vi "IHL_Wait for Start Pos Helper.vi"(8 "error in (no error)":errorcluster, 10 "Inspect Helper Loop Data":T1={"IHL State"=enum."Init", "Timeout"=0, "Loop Count"=0, "Start Sample No."=0, "Collecting Data"=FALSE, "No. Samples"=0, "Success Flag"=FALSE, "Inspect Status "={"Ready"=FALSE, "Inspecting"=FALSE, "Cancel"=FALSE}, "Status"=0, "Encoder Count"=0, "PosToStartScan"=50800, "ScanLength"=50800, "MaxSamples"=50800, "PosToEndScan"=0, "Host SampleData"=refnum, "data value reference"=refnum, "Block Cnt notifier out"=refnum, "EventLog"=refnum}, 11 "Message Queue in":refnum<class "Delacor_lib_QMH_Message Queue.lvclass">) -> (0 "error out":errorcluster, 2 "Inspect Helper Loop Data out":T1={"IHL State"=enum."Init", "Timeout"=0, "Loop Count"=0, "Start Sample No."=0, "Collecting Data"=FALSE, "No. Samples"=0, "Success Flag"=FALSE, "Inspect Status "={"Ready"=FALSE, "Inspecting"=FALSE, "Cancel"=FALSE}, "Status"=0, "Encoder Count"=0, "PosToStartScan"=50800, "ScanLength"=50800, "MaxSamples"=50800, "PosToEndScan"=0, "Host SampleData"=refnum, "data value reference"=refnum, "Block Cnt notifier out"=refnum, "EventLog"=refnum})   [LabVIEW 2015, in "Tool Module.lvlib"]
uses:
  Tool Module.lvlib
  _IHL Data Cluster--typedef.ctl
  Event Logger Library/Event Log/EventLog.lvclass
  _IHL SM Enum--typedef.ctl
  _IHL Status Update Cluster--typedef.ctl
  _Sample Data Rtn Cluster--typedef.ctl
  <vilib>/Delacor/Delacor QMH/Libraries/Message Queue_class/Delacor_lib_QMH_Message Queue.lvclass
  <vilib>/Delacor/Delacor QMH/Libraries/Message Queue_class/Delacor_lib_QMH_Message Queue.lvclass/Delacor_lib_QMH_Message Queue.ctl
  <vilib>/Delacor/Delacor QMH/Libraries/Message Queue_class/Delacor_lib_QMH_Enqueue Message (Single).vi
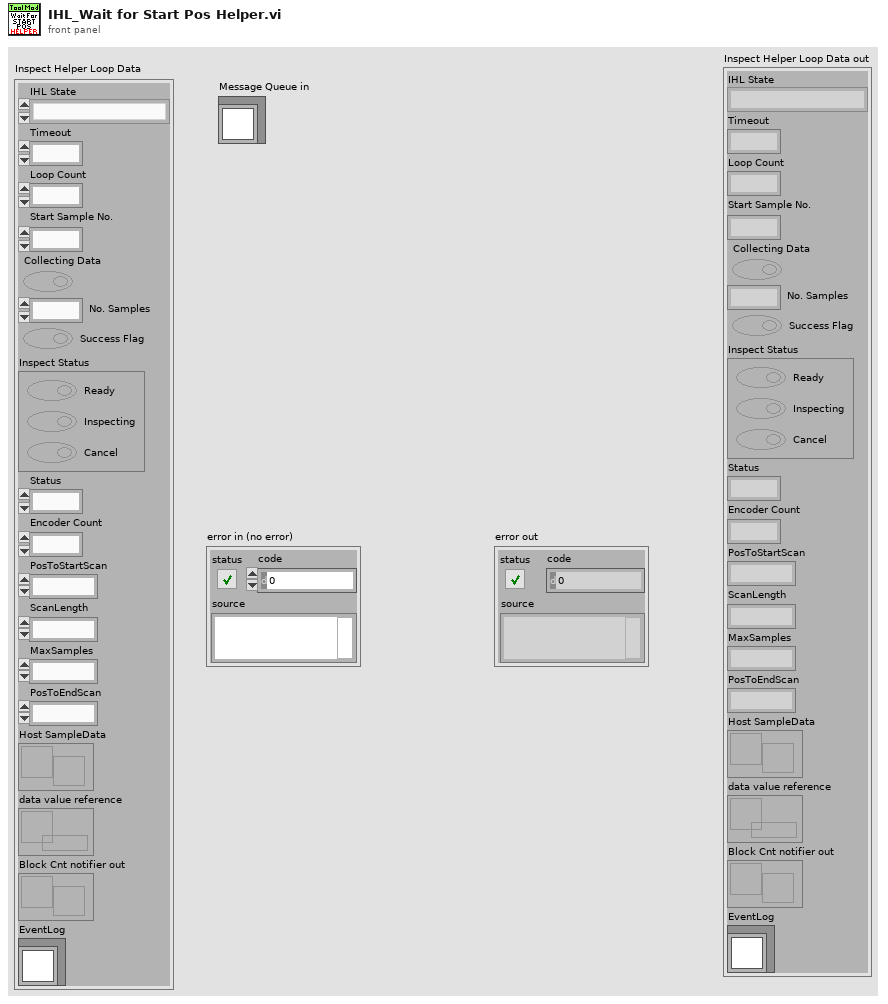
[diagram p1: front panel]
types:
  T1 = typedef "Tool Module.lvlib/_IHL Data Cluster--typedef.ctl" = cluster{"IHL State":T2, "Timeout":i32, "Loop Count":i32, "Start Sample No.":u32, "Collecting Data":bool, "No. Samples":i32, "Success Flag":bool, "Inspect Status ":T3, "Status":u16, "Encoder Count":i32, "PosToStartScan":i32, "ScanLength":i32, "MaxSamples":i32, "PosToEndScan":i32, "Host SampleData":refnum<notifier>, "data value reference":refnum<data-value>, "Block Cnt notifier out":refnum<notifier>, "EventLog":refnum<class "EventLog.lvclass">}
  T2 = typedef "Tool Module.lvlib/_IHL SM Enum--typedef.ctl" = enum16{"Init", "Set Motion Speed", "Move To Scan Start", "Wait for Motion Out", "Wait for Start Pos", "Inspect: START", "Wait for Motion IN", "Wait for Inspect Range", "Inspecting", "Inspect: STOP"}
  T3 = typedef "Tool Module.lvlib/_IHL Status Update Cluster--typedef.ctl" = cluster{"Ready":bool, "Inspecting":bool, "Cancel":bool}
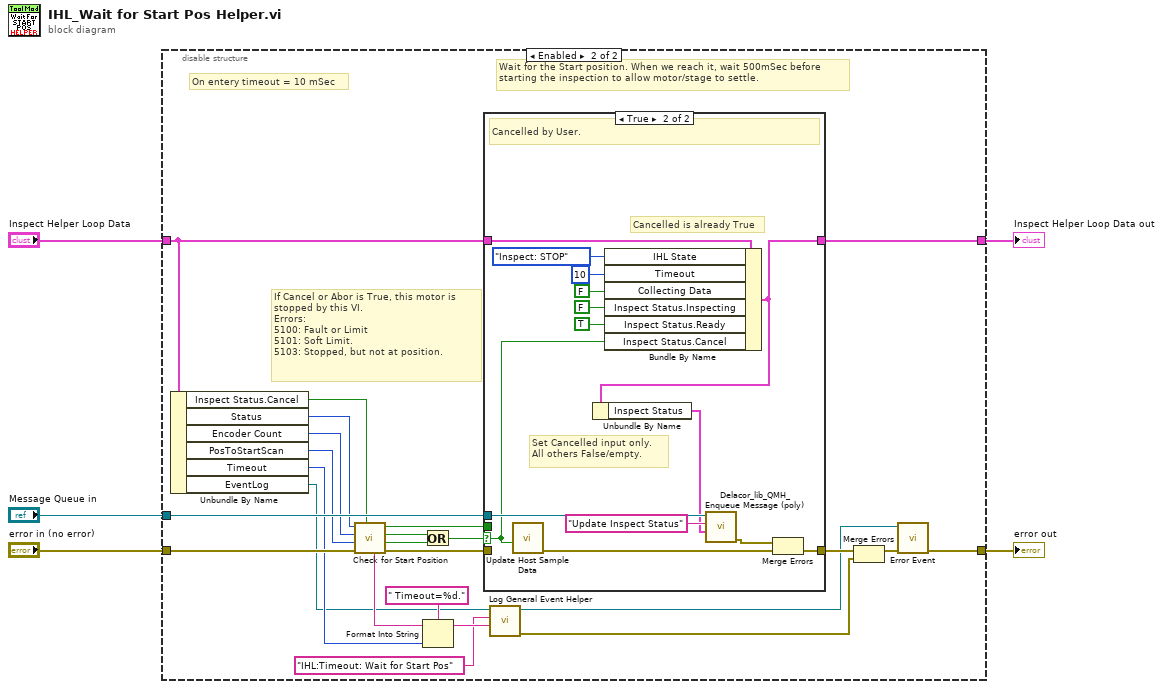
[diagram p0: block diagram]
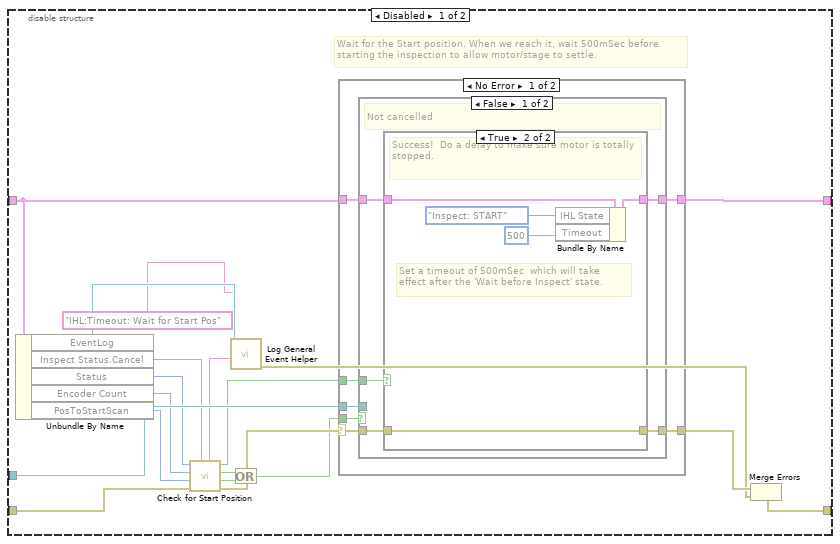
[diagram p2: hidden frame]
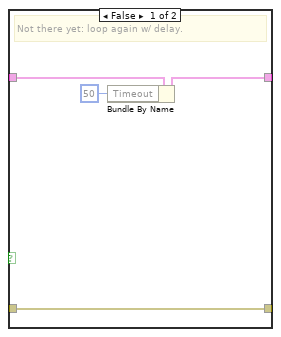
[diagram p3: hidden frame]
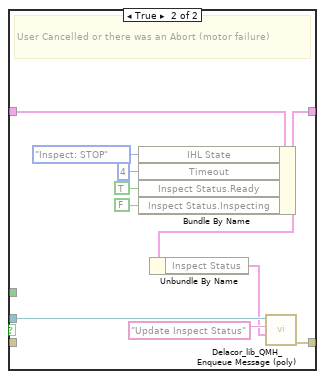
[diagram p4: hidden frame]
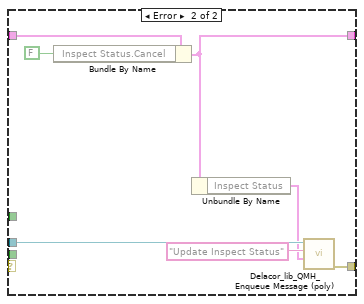
[diagram p5: hidden frame]
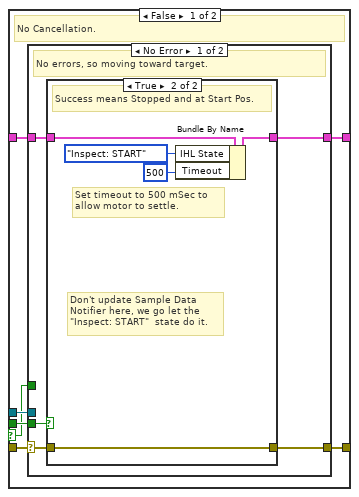
[diagram p6: hidden frame]
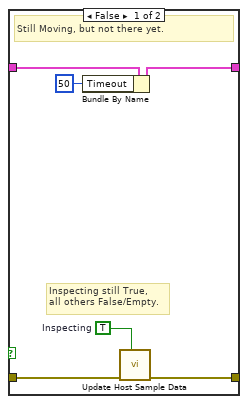
[diagram p7: hidden frame]
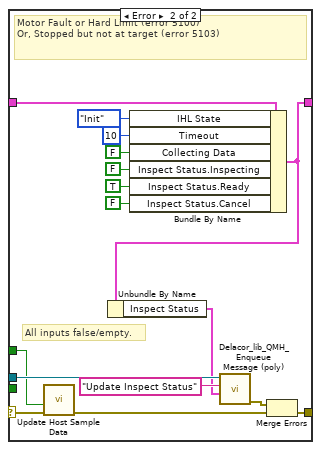
[diagram p8: hidden frame]
diagram:
  n1 = disable-structure shown="Enabled" {
    disable-tunnel: "Message Queue in" -> [w23 w80]
    disable-tunnel: "error in (no error)" -> [w18 w78]
    disable-tunnel: "Inspect Helper Loop Data" -> [w17 w81]
    disable-tunnel: [w11 w82] -> w2
    disable-tunnel: [w7 w72] -> w1
    frame Disabled {
      # "Wait for the Start position. When we reach it, wait 500mSec before starting the inspection to allow motor/stage to settle."
      n2 = Unbundle By Name(w17) -> ("EventLog"=w10:refnum<class "EventLog.lvclass">, "Inspect Status.Cancel"=w22:bool, "Status"=w21:u16, "Encoder Count"=w20:i32, "PosToStartScan"=w19:i32)
      n3 = call "Check for Start Position.vi"("Cancel Inspect"=w22, "error in (no error)"=w18, "Target Encdr Pos."=w19, "Cur Encoder Value"=w20, "Status Byte"=w21) -> ("error out"=w24:errorcluster, "Aborted"=w16:bool, "Cancelled"=w15:bool, "Success"=w13:bool, "Log String out"=w9:string)  [unwired: 2 in]
      n4 = call "Log General Event Helper.vi"("Payload"=w9, "State Info"="IHL:Timeout: Wait for Start Pos", "EventLog in"=w10) -> ("error out"=w6:errorcluster)  [unwired: 7 in, 1 out]
      n5 = Or(x=w15, y=w16) -> (x .or. y?=w14:bool)
      n6 = case shown="No Error" w24 {
        selector: w24 -> [w25 _]
        tunnel: [w31 w60] -> w12
        tunnel: w23 -> [w30 w59]
        tunnel: w17 -> [w29 w62]
        tunnel: [w28 w57] -> w11
        tunnel: w14 -> [w27 _]
        tunnel: w13 -> [w26 _]
        frame No Error {
          n7 = case shown="False" w27 {
            tunnel: [w32 w55] -> w31
            tunnel: w30 -> [_ w54]
            tunnel: w29 -> [w34 w52]
            tunnel: [w33 w51] -> w28
            tunnel: w26 -> [w36 _]
            tunnel: w25 -> [w35 _]
            frame False {
              # "Not cancelled"
              n8 = case shown="True" w36 {
                tunnel: w35 -> [w37 w41]
                tunnel: w34 -> [w40 w45]
                tunnel: [w39 w44] -> w33
                tunnel: [w37 w41] -> w32
                frame False {
                  # "Not there yet: loop again w/ delay."
                  n9 = Bundle By Name(cluster=w40, "Timeout"=50) -> (w39:T1)
                }
                frame True {
                  # "Set a timeout of 500mSec  which will take effect after the 'Wait before Inspect' state."
                  # "Success!  Do a delay to make sure motor is totally stopped."
                  n10 = Bundle By Name(cluster=w45, "IHL State"=_IHL_SM_Enum--typedef."Inspect: START" ("Inspect State"), "Timeout"=500) -> (w44:T1)
                }
              }
            }
            frame True {
              # "User Cancelled or there was an Abort (motor failure)"
              n11 = Bundle By Name(cluster=w52, "IHL State"=_IHL_SM_Enum--typedef."Inspect: STOP" ("Inspect State"), "Timeout"=4, "Inspect Status.Ready"=TRUE ("Inspect Status .Ready"), "Inspect Status.Inspecting"=FALSE ("Inspect Status .Inspecting")) -> (w51:T1)
              n12 = Unbundle By Name(w51) -> ("Inspect Status"=w48:T3)
              n13 = call-poly <vilib>:"Delacor_lib_QMH_Enqueue Message (poly).vi"("Message Data"=w48, "Message"="Update Inspect Status", "Message Queue in"=w54) -> ("error out"=w55:errorcluster)  [unwired: 7 in, 1 out]
            }
          }
        }
        frame Error {
          n14 = Bundle By Name(cluster=w62, "Inspect Status.Cancel"=FALSE ("Inspect Status .Cancel")) -> (w57:T1)
          n15 = Unbundle By Name(w57) -> ("Inspect Status"=w56:T3)
          n16 = call-poly <vilib>:"Delacor_lib_QMH_Enqueue Message (poly).vi"("Message Data"=w56, "Message"="Update Inspect Status", "Message Queue in"=w59) -> ("error out"=w60:errorcluster)  [unwired: 7 in, 1 out]
        }
      }
      n17 = Merge Errors(w12, w6) -> (w7:errorcluster)
    }
    frame Enabled {
      # "If Cancel or Abor is True, this motor is stopped by this VI.\nErrors: \n5100: Fault or Limit\n5101: Soft Limit. \n5103: Stopped, but not at position."
      # "On entery timeout = 10 mSec"
      # "Wait for the Start position. When we reach it, wait 500mSec before starting the inspection to allow motor/stage to settle."
      n18 = Unbundle By Name(w81) -> ("Inspect Status.Cancel"=w66:bool, "Status"=w67:u16, "Encoder Count"=w77:i32, "PosToStartScan"=w76:i32, "Timeout"=w69:i32, "EventLog"=w68:refnum<class "EventLog.lvclass">)
      n19 = call "Check for Start Position.vi"("Cancel Inspect"=w66, "error in (no error)"=w78, "Target Encdr Pos."=w76, "Cur Encoder Value"=w77, "Status Byte"=w67) -> ("error out"=w75:errorcluster, "Aborted"=w65:bool, "Cancelled"=w64:bool, "Success"=w74:bool, "Log String out"=w70:string)  [unwired: 2 in]
      n20 = Or(x=w64, y=w65) -> (x .or. y?=w63:bool)
      n21 = Format Into String(format string=" Timeout=%d.", initial string=w70, w69) -> (resulting string=w85:string)  [unwired: 1 in, 1 out]
      n22 = case shown="True" w63 {
        selector: w63 -> [w87 w126]
        tunnel: [w92 w131] -> w82
        tunnel: w81 -> [w93 w139]
        tunnel: w80 -> [w89 w133]
        tunnel: [w90 w128] -> w79
        tunnel: w75 -> [w91 _]
        tunnel: w74 -> [w88 _]
        frame False {
          # "No Cancellation."
          n23 = case shown="No Error" w91 {
            selector: w91 -> [w95 w114]
            tunnel: w93 -> [w97 w125]
            tunnel: [w96 w118] -> w92
            tunnel: [w94 w111] -> w90
            tunnel: w89 -> [_ w120]
            tunnel: w88 -> [w98 _]
            tunnel: w87 -> [_ w113]
            frame No Error {
              # "No errors, so moving toward target."
              n24 = case shown="True" w98 {
                tunnel: [w103 w108] -> w96
                tunnel: w97 -> [w104 w109]
                tunnel: w95 -> [w100 w105]
                tunnel: [w99 w105] -> w94
                frame False {
                  w101 = TRUE  # Inspecting
                  # "Inspecting still True,\nall others False/Empty."
                  # "Still Moving, but not there yet."
                  n25 = Bundle By Name(cluster=w104, "Timeout"=50) -> (w103:T1)
                  n26 = call "Update Host Sample Data.vi"("Inspecting"=w101, "error in (no error)"=w100) -> ("error out"=w99:errorcluster)  [unwired: 9 in]
                }
                frame True {
                  # "Don't update Sample Data Notifier here, we go let the  \"Inspect: START\"  state do it."
                  # "Set timeout to 500 mSec to allow motor to settle."
                  # "Success means Stopped and at Start Pos."
                  n27 = Bundle By Name(cluster=w109, "IHL State"=_IHL_SM_Enum--typedef."Inspect: START" ("Inspect State"), "Timeout"=500) -> (w108:T1)
                }
              }
            }
            frame Error {
              # "All inputs false/empty."
              # "Motor Fault or Hard Limit (error 5100)\nOr, Stopped but not at target (error 5103)"
              n28 = call "Update Host Sample Data.vi"("error in (no error)"=w114, "Cancelled"=w113) -> ("error out"=w110:errorcluster)  [unwired: 9 in]
              n29 = Bundle By Name(cluster=w125, "IHL State"=_IHL_SM_Enum--typedef."Init" ("Inspect State"), "Timeout"=10, "Collecting Data"=FALSE, "Inspect Status.Inspecting"=FALSE ("Inspect Status .Inspecting"), "Inspect Status.Ready"=TRUE ("Inspect Status .Ready"), "Inspect Status.Cancel"=FALSE ("Inspect Status .Cancel")) -> (w118:T1)
              n30 = Unbundle By Name(w118) -> ("Inspect Status"=w117:T3)
              n31 = call-poly <vilib>:"Delacor_lib_QMH_Enqueue Message (poly).vi"("Message Data"=w117, "Message"="Update Inspect Status", "Message Queue in"=w120) -> ("error out"=w112:errorcluster)  [unwired: 7 in, 1 out]
              n32 = Merge Errors(w112, w110) -> (w111:errorcluster)
            }
          }
        }
        frame True {
          # "Set Cancelled input only. All others False/empty."
          # "Cancelled is already True"
          # "Cancelled by User."
          n33 = call "Update Host Sample Data.vi"("Cancelled"=w126) -> ("error out"=w129:errorcluster)  [unwired: 10 in]
          n34 = Bundle By Name(cluster=w139, "IHL State"=_IHL_SM_Enum--typedef."Inspect: STOP" ("Inspect State"), "Timeout"=10, "Collecting Data"=FALSE, "Inspect Status.Inspecting"=FALSE ("Inspect Status .Inspecting"), "Inspect Status.Ready"=TRUE ("Inspect Status .Ready"), "Inspect Status.Cancel"=w126) -> (w131:T1)
          n35 = Unbundle By Name(w131) -> ("Inspect Status"=w130:T3)
          n36 = call-poly <vilib>:"Delacor_lib_QMH_Enqueue Message (poly).vi"("Message Data"=w130, "Message"="Update Inspect Status", "Message Queue in"=w133) -> ("error out"=w127:errorcluster)  [unwired: 7 in, 1 out]
          n37 = Merge Errors(w127, w129) -> (w128:errorcluster)
        }
      }
      n38 = call "Log General Event Helper.vi"("Payload"=w85, "State Info"="IHL:Timeout: Wait for Start Pos", "EventLog in"=w68) -> ("error out"=w83:errorcluster, "EventLog out"=w71:refnum<class "EventLog.lvclass">)  [unwired: 7 in]
      n39 = Merge Errors(w79, w83) -> (w73:errorcluster)
      n40 = call "Error Event.vi"("error in (no error)"=w73, "EventLog ref"=w71) -> ("error out"=w72:errorcluster)  [unwired: 8 in, 1 out]
    }
  }
  "error out" <- w1
  "Inspect Helper Loop Data out" <- w2
